vi "Tester Client.vi"() -> ()   [LabVIEW 2017]
uses:
  <vilib>/ActorFramework/Message Enqueuer/Message Enqueuer.lvclass/Message Enqueuer.ctl
  Actors/WebSocket Client/WebSocket Client Messages/Send Message Msg/Send Message Msg.lvclass/Send Message Msg.ctl
  <vilib>/ActorFramework/Message Enqueuer/Enqueue.vi
  Actors/WebSocket Client/WebSocket Client/WebSocket Client.lvclass
  Applications/National Instruments/LabVIEW 2017 64-bit/vi.lib/ActorFramework/Actor/Actor.lvclass
  <vilib>/ActorFramework/Stop Msg/Stop Msg.lvclass
  Applications/National Instruments/LabVIEW 2017 64-bit/vi.lib/ActorFramework/Message/Message.lvclass
  Actors/WebSocket Client/WebSocket Client Messages/Send Message Msg/Send Message Msg.lvclass
  <vilib>/ActorFramework/Message Priority Queue/Priority Enqueue.vi
  <vilib>/ActorFramework/Actor/Actor.lvclass
panel:
  in  "client":bool
  in  "String":string
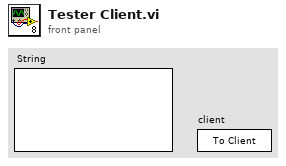
[diagram p1: front panel]
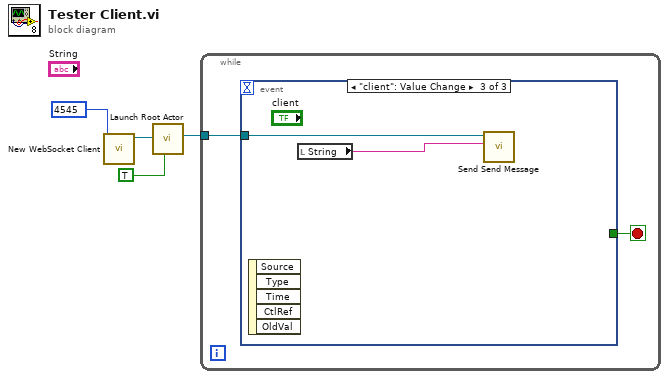
[diagram p0: block diagram]
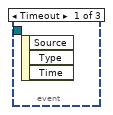
[diagram p2: hidden frame]
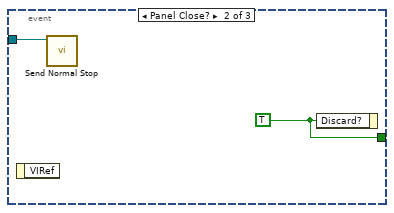
[diagram p3: hidden frame]
diagram:
  n1 = call "New WebSocket Client.vi"("Port"=u16 4545) -> ("WebSocket Client out"=w2:refnum<class "WebSocket Client.lvclass">)  [unwired: 9 in, 1 out]
  n2 = call <vilib>:"Launch Root Actor.vi"("Open Actor Core front panel? (F)"=TRUE, "Actor"=w2) -> ("Actor's Enqueuer"=w3:refnum<class "Message Enqueuer.lvclass">)  [unwired: 8 in, 1 out]
  n3 = while {
    tunnel: w3 -> [w5]
    stop <- w6 stop-if-true
    n4 = event shown="[2] \"client\": Value Change" {
      selector: _ -> [_ _ _]
      dyn-events: _ -> [_ _ _]
      timeout: _ -> [_ _ _]
      tunnel: [_ w8 _] -> w6
      tunnel: w5 -> [_ w7 w10]
      event Timeout {
        n5 = event-data() -> ()  [unwired: 1 in, 3 out]
      }
      event Panel Close? {
        w8 = TRUE ("Discard?")
        n6 = event-data() -> ()  [unwired: 1 in, 1 out]
        n7 = call <vilib>:"Send Normal Stop.vi"("Message Enqueuer"=w7) -> ()  [unwired: 10 in, 1 out]
        n8 = event-data("Discard?"=w8) -> ()  [unwired: 1 in, 1 out]
      }
      event "client": Value Change {
        n9 = event-data() -> ()  [unwired: 1 in, 5 out]
        n10 = local read "String"() -> (w9:string)
        n11 = call "Send Send Message.vi"("Message"=w9, "Message Enqueuer in"=w10) -> ()  [unwired: 8 in, 2 out]
      }
    }
  }
